vi "Remove Transfer.vi"(8 "error in (no error)":errorcluster, 10 "ID":string, 11 "dsf refnum":T1) -> (0 "error out":errorcluster, 3 "dsf refnum out":T1, 4 "exists?":bool)   [LabVIEW 2017, in "Data Sharing Framework Core.lvlib" / "Data Sharing Framework Configuration.lvlib"]
doc: "Removes a section from the configuration data identified by <B>dsf refnum</B>."
uses:
  Data Sharing Framework Configuration.lvlib
  Controls/DSF Config Data RefNum.ctl
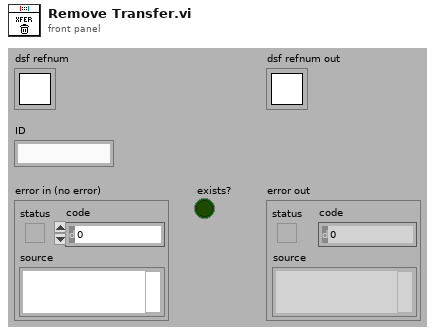
[diagram p1: front panel]
types:
  T1 = typedef "Data Sharing Framework Core.lvlib/Data Sharing Framework Configuration.lvlib/DSF Config Data RefNum.ctl" = refnum<k1>
  T2 = typedef "Data Sharing Framework Core.lvlib/Data Sharing Framework Configuration.lvlib/DSF Configuration Reference.ctl" = refnum<data-value>
  T3 = typedef "Data Sharing Framework Core.lvlib/Data Sharing Framework Configuration.lvlib/Internal.DSF Configuration.ctl" = cluster{"dsfversion":T4, "version":T4, "plugins":T5[], "groups":T8[], "transfers":T10[], "channels":T12[], "settings":T14[]}
  T4 = typedef "Data Sharing Framework Core.lvlib/Data Sharing Framework Configuration.lvlib/DSF Version Info.ctl" = cluster{"major":u32, "minor":u32, "fix":u32, "build":string}
  T5 = typedef "Data Sharing Framework Core.lvlib/Data Sharing Framework Configuration.lvlib/Internal.DSF Plugin with ID.ctl" = cluster{"id":string, "values":T6}
  T6 = typedef "Data Sharing Framework Core.lvlib/Data Sharing Framework Configuration.lvlib/Internal.DSF Plugin Info.ctl" = cluster{"type":string, "timing":T7, "group ids":string[], "settings id":string}
  T7 = typedef "Data Sharing Framework Core.lvlib/Data Sharing Framework Configuration.lvlib/DSF Timing Info.ctl" = cluster{"priority":u64, "decimation":u64, "offset":u64}
  T8 = typedef "Data Sharing Framework Core.lvlib/Data Sharing Framework Configuration.lvlib/Internal.DSF Group with ID.ctl" = cluster{"id":string, "values":T9}
  T9 = typedef "Data Sharing Framework Core.lvlib/Data Sharing Framework Configuration.lvlib/Internal.DSF Group Info.ctl" = cluster{"direction":i32, "timing":T7, "transfer ids":string[], "settings id":string}
  T10 = typedef "Data Sharing Framework Core.lvlib/Data Sharing Framework Configuration.lvlib/Internal.DSF Transfer with ID.ctl" = cluster{"id":string, "values":T11}
  T11 = typedef "Data Sharing Framework Core.lvlib/Data Sharing Framework Configuration.lvlib/Internal.DSF Transfer Info.ctl" = cluster{"byte order":i32, "channel ids":string[], "settings id":string}
  T12 = typedef "Data Sharing Framework Core.lvlib/Data Sharing Framework Configuration.lvlib/Internal.DSF Channel with ID.ctl" = cluster{"id":string, "values":T13}
  T13 = typedef "Data Sharing Framework Core.lvlib/Data Sharing Framework Configuration.lvlib/Internal.DSF Channel Info.ctl" = cluster{"count":u64, "buffer offset":u64, "data type":i32, "settings id":string}
  T14 = typedef "Data Sharing Framework Core.lvlib/Data Sharing Framework Configuration.lvlib/Internal.DSF Settings with ID.ctl" = cluster{"id":string, "values":T15}
  T15 = typedef "Data Sharing Framework Core.lvlib/Data Sharing Framework Configuration.lvlib/Internal.DSF Settings Info.ctl" = cluster{"key":string, "value":string}[]
  T16 = cluster{"dsf configuration":T3, "path":path, "dirty":bool}
  T17 = typedef "Data Sharing Framework Core.lvlib/Data Sharing Framework Configuration.lvlib/DSF Config Data.ctl" = cluster{"dsf configuration":T3, "path":path, "dirty":bool}
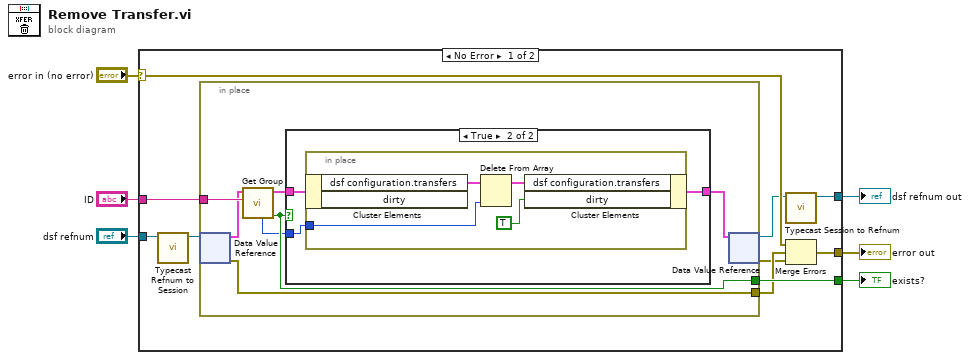
[diagram p0: block diagram]
diagram:
  n1 = case shown="No Error" "error in (no error)" {
    selector: "error in (no error)" -> [w14 w33]
    tunnel: [w9 w33] -> w1
    tunnel: [w15 w32] -> w3
    tunnel: "dsf refnum" -> [w16 w32]
    tunnel: "ID" -> [w13 _]
    tunnel: [w12 _] -> w2
    frame No Error {
      n2 = call "Typecast Refnum to Session.vi"("dsf refnum in"=w16) -> ("DSF Configuration Session out"=w11:T2)  [unwired: 10 out]
      n3 = in-place {
        in-place-border: w13 -> [w23]
        in-place-border: [w22] -> w12
        in-place-border: [w17] -> w8
        n4 = in-place-dvr #1(w11) -> (w19:T16, w17:errorcluster)
        n5 = call "Get Group.vi"("id"=w23, "DSF Configuration in"=w19) -> ("exists?"=w22:bool, "DSF Configuration out"=w21:T17, "index"=w20:i32)  [unwired: 6 in, 1 out]
        n6 = case shown="True" w22 {
          tunnel: [w24 w27] -> w18
          tunnel: w20 -> [_ w26]
          tunnel: w21 -> [w24 w25]
          frame False {
          }
          frame True {
            n7 = in-place {
              in-place-border: w26 -> [w31]
              n8 = in-place-cluster #2(w25) -> ("dsf configuration.transfers"=w30:T10[])  [unwired: 1 out]
              n9 = Delete From Array(array=w30, index=w31) -> (array with subset deleted=w29:T10[])  [unwired: 1 in, 1 out]
              n10 = in-place-cluster #2("dsf configuration.transfers"=w29, "dirty"=TRUE) -> (w27:T17)
            }
          }
        }
        n11 = in-place-dvr #1(w18) -> (w10:T2, w7:errorcluster)
      }
      n12 = call "Typecast Session to Refnum.vi"("DSF Configuration Session in"=w10) -> ("dsf refnum out"=w15:T1)  [unwired: 10 out]
      n13 = Merge Errors(w14, w8, w7) -> (w9:errorcluster)
    }
    frame Error {
    }
  }
  "error out" <- w1
  "exists?" <- w2
  "dsf refnum out" <- w3
